vi "value to ring (PayloadGenerationMode).vi"(11 "value":string) -> (3 "PayloadGenerationMode":i32(ring) items=["FDX_TX_FRAME_PGM_USER", "FDX_TX_FRAME_PGM_IP_PART", "FDX_TX_FRAME_PBM_UDP", "FDX_TX_FRAME_PGM_IP_PART_TT", "FDX_TX_FRAME_PGM_IP_FULL", "FDX_TX_FRAME_PGM_IP_FULL_TT"])   [LabVIEW 2020, in "AIM ARINC 664 Import.lvlib"]
uses:
  AIM ARINC 664 Import.lvlib
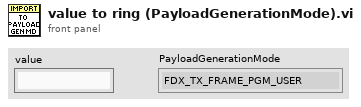
[diagram p1: front panel]
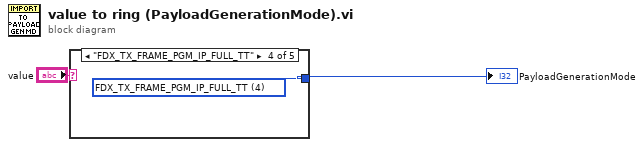
[diagram p0: block diagram]
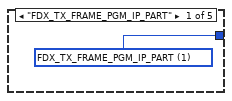
[diagram p2: hidden frame]
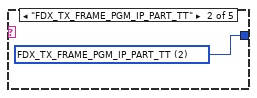
[diagram p3: hidden frame]
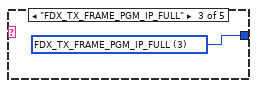
[diagram p4: hidden frame]
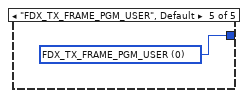
[diagram p5: hidden frame]
diagram:
  n1 = case shown="\"FDX_TX_FRAME_PGM_IP_FULL_TT\"" "value" {
    tunnel: [w3 w4 w5 w6 w7] -> w1
    frame "FDX_TX_FRAME_PGM_IP_PART" {
      w3 = 1 items=["FDX_TX_FRAME_PGM_USER", "FDX_TX_FRAME_PGM_IP_PART", "FDX_TX_FRAME_PGM_IP_PART_TT", "FDX_TX_FRAME_PGM_IP_FULL", "FDX_TX_FRAME_PGM_IP_FULL_TT"] ("PayloadGenerationMode")
    }
    frame "FDX_TX_FRAME_PGM_IP_PART_TT" {
      w4 = 2 items=["FDX_TX_FRAME_PGM_USER", "FDX_TX_FRAME_PGM_IP_PART", "FDX_TX_FRAME_PGM_IP_PART_TT", "FDX_TX_FRAME_PGM_IP_FULL", "FDX_TX_FRAME_PGM_IP_FULL_TT"] ("PayloadGenerationMode")
    }
    frame "FDX_TX_FRAME_PGM_IP_FULL" {
      w5 = 3 items=["FDX_TX_FRAME_PGM_USER", "FDX_TX_FRAME_PGM_IP_PART", "FDX_TX_FRAME_PGM_IP_PART_TT", "FDX_TX_FRAME_PGM_IP_FULL", "FDX_TX_FRAME_PGM_IP_FULL_TT"] ("PayloadGenerationMode")
    }
    frame "FDX_TX_FRAME_PGM_IP_FULL_TT" {
      w6 = 4 items=["FDX_TX_FRAME_PGM_USER", "FDX_TX_FRAME_PGM_IP_PART", "FDX_TX_FRAME_PGM_IP_PART_TT", "FDX_TX_FRAME_PGM_IP_FULL", "FDX_TX_FRAME_PGM_IP_FULL_TT"] ("PayloadGenerationMode")
    }
    frame "FDX_TX_FRAME_PGM_USER", Default {
      w7 = 0 items=["FDX_TX_FRAME_PGM_USER", "FDX_TX_FRAME_PGM_IP_PART", "FDX_TX_FRAME_PGM_IP_PART_TT", "FDX_TX_FRAME_PGM_IP_FULL", "FDX_TX_FRAME_PGM_IP_FULL_TT"] ("PayloadGenerationMode")
    }
  }
  "PayloadGenerationMode" <- w1
